vi "Host - Refresh All.vi"(8 "error in (no error)":errorcluster, 11 "serverName":string="10.0.18.244") -> (0 "error out":errorcluster, 3 "serverName":string="10.0.18.244")   [LabVIEW 2019, in "Scan Engine Custom Device.lvlib"]
uses:
  Scan Engine Custom Device.lvlib
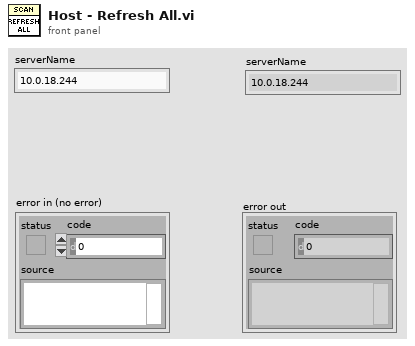
[diagram p1: front panel]
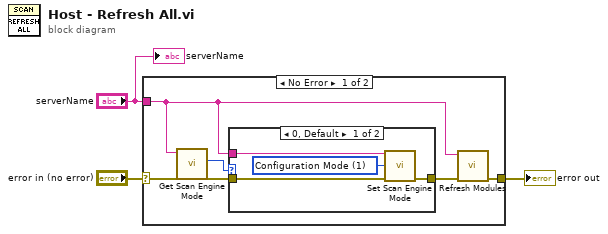
[diagram p0: block diagram]
diagram:
  n1 = case shown="No Error" "error in (no error)" {
    selector: "error in (no error)" -> [w7 w15]
    tunnel: "serverName" -> [w5 _]
    tunnel: [w4 w15] -> w1
    frame No Error {
      n2 = call <vilib>:"Get Scan Engine Mode.vi"("error in (no error)"=w7, "target address (localhost)"=w5) -> ("error out"=w9:errorcluster, "mode"=w8:i32)  [unwired: 8 in]
      n3 = case shown="0, Default" w8 {
        tunnel: w5 -> [w12 _]
        tunnel: w9 -> [w11 w14]
        tunnel: [w10 w14] -> w6
        frame 0, Default {
          w13 = 1 items=["Configuration Mode"=1, "Active Mode"=2] ("mode (Active Mode)")
          n4 = call <vilib>:"Set Scan Engine Mode.vi"("target address (localhost)"=w12, "mode (Active Mode)"=w13, "error in (no error)"=w11) -> ("error out"=w10:errorcluster)  [unwired: 12 in]
        }
        frame 1 {
        }
      }
      n5 = call <vilib>:"Refresh Modules.vi"("error in (no error)"=w6, "target address (localhost)"=w5) -> ("error out"=w4:errorcluster)  [unwired: 9 in]
    }
    frame Error {
    }
  }
  "error out" <- w1
  "serverName" <- "serverName"
